vi "Agilent 3446X Series Acquire Single in loop.vi"() -> ()   [LabVIEW 2014]
doc: "This example shows how to configure a measurement and take a reading."
uses:
  DAQ LabVIEW/ISCOOL Agilent readout/Public/Data/Read (Single Point).vi
  DAQ LabVIEW/ISCOOL Agilent readout/Agilent 3446X Series.lvlib
panel:
  in  "Sample rate":dbl
  in  "stop":bool
  in  "VISA resource name":refnum<visa-resource-name>
  in  "Manual Range (1)":dbl=1.0
  in  "Auto Range (T: Enable)":bool=TRUE
  in  "Absolute Resolution (1E-6)":dbl=1e-06
  in  "Measurement Function (10: Voltage DC)":i32(ring)=10 items=["Continuity", "Current AC", "Current DC", "Diode", "Frequency", "Resistance 4-wire", "Period", "Resistance 2-wire", "Temperature", "Voltage AC", "Voltage DC", "Voltage DC Ratio"]
  out "Measurement":dbl
  # "(c) 2013 National Instruments.  ALL RIGHTS RESERVED."
  # "TCPIP0::A-34461A-06386::inst0::INSTR"
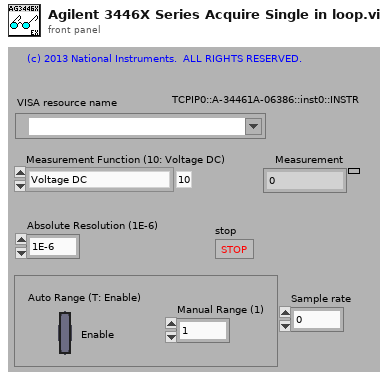
[diagram p1: front panel]
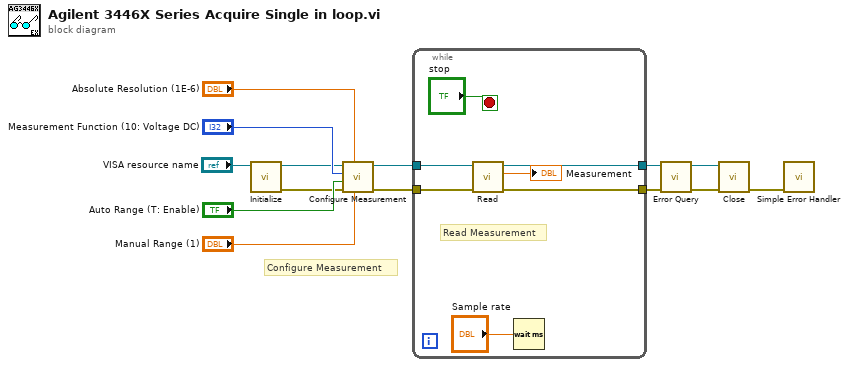
[diagram p0: block diagram]
diagram:
  # "Configure Measurement"
  n1 = call "Initialize.vi"("VISA resource name"="VISA resource name") -> ("error out"=w9:errorcluster, "VISA resource name out"=w8:refnum<visa-resource-name>)  [unwired: 4 in, 5 out]
  n2 = call "Configure Measurement.vi"("Manual Range (1)"="Manual Range (1)", "Absolute Resolution (1E-6)"="Absolute Resolution (1E-6)", "error in (no error)"=w9, "Auto Range (T: Enable)"="Auto Range (T: Enable)", "Measurement Function (10: Voltage DC)"="Measurement Function (10: Voltage DC)", "VISA resource name"=w8) -> ("error out"=w6:errorcluster, "VISA resource name out"=w7:refnum<visa-resource-name>)  [unwired: 4 out]
  n3 = while {
    tunnel: w7 -> [w19]
    tunnel: w6 -> [w18]
    tunnel: [w17] -> w2
    tunnel: [w16] -> w1
    stop <- "stop" stop-if-true
    # "Read Measurement"
    n4 = call-poly "Read.vi"("error in (no error)"=w18, "VISA resource name"=w19) -> ("error out"=w16:errorcluster, "Measurement"=→"Measurement":dbl, "VISA resource name out"=w17:refnum<visa-resource-name>)  [unwired: 7 out]
    n5 = Wait (ms)(milliseconds to wait="Sample rate") -> ()  [unwired: 1 out]
  }
  n6 = call "Error Query.vi"("error in (no error)"=w1, "VISA resource name"=w2) -> ("error out"=w3:errorcluster, "VISA resource name out"=w4:refnum<visa-resource-name>)  [unwired: 8 out]
  n7 = call "Close.vi"("error in (no error)"=w3, "VISA resource name"=w4) -> ("error out"=w5:errorcluster)  [unwired: 9 out]
  n8 = call <vilib>:"Simple Error Handler.vi"("error in (no error)"=w5) -> ()  [unwired: 1 in, 8 out]
